vi "Subversion Get Status.vi"() -> (0 "error out":errorcluster, 1 "Working copy URL":string, 2 "Last \"Updated\" Date?":string, 3 "SVN Status":string)   [LabVIEW 2023]
uses:
  <vilib>/Utility/error.llb/Trim Whitespace One-Sided.vi
  <vilib>/regexp/Match Regular Expression.xnode
panel:
  out "Inhomogeneous revision?":bool
  out "Revision range if inhomogeneous":string
  out "Working copy uncommitted?":bool
  out "All Changed Files":string="0"
  out "Last Revision Different?":bool
  out "Last Revision":i32
  out "Revision":i32
  out "svn info":string
  out "Application Top-Level":path
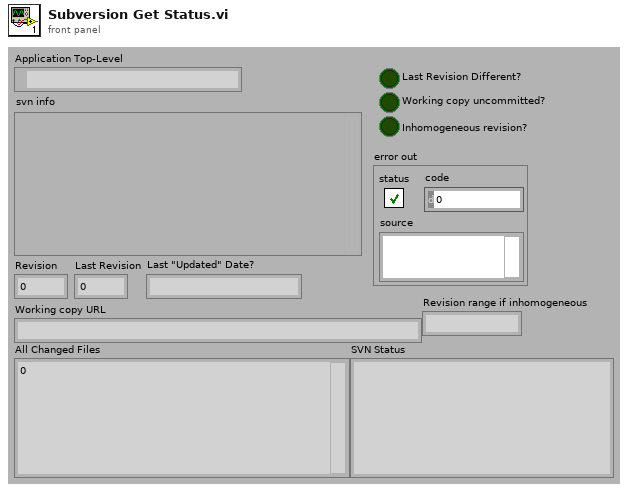
[diagram p1: front panel]
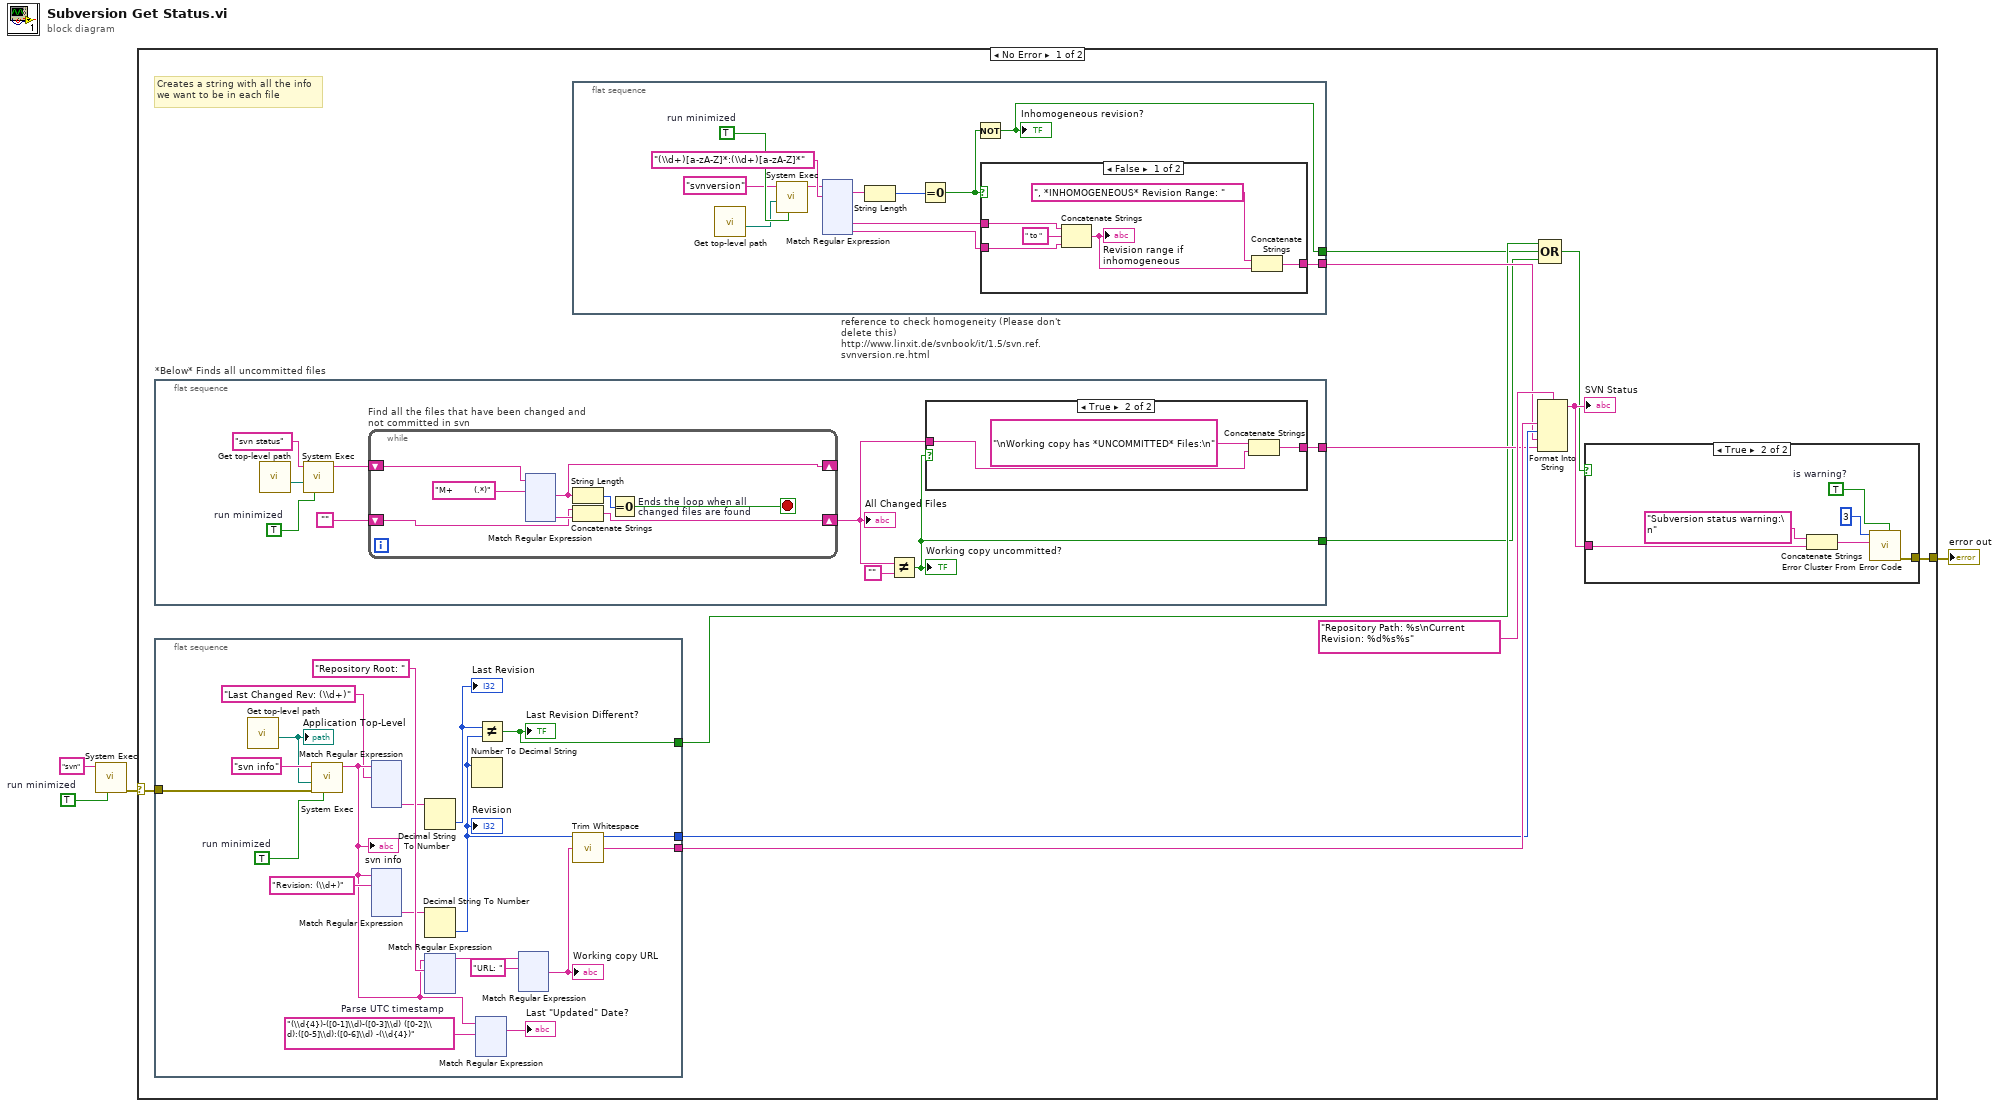
[diagram p0: block diagram]
diagram:
  w2 = TRUE  # run minimized
  n1 = call <vilib>:"System Exec.vi"("run minimized? (F)"=w2, "command line"="svn") -> ("error out"=w4:errorcluster)  [unwired: 4 in, 5 out]
  n2 = case shown="No Error" w4 {
    selector: w4 -> [w16 _]
    tunnel: [w5 _] -> w1
    frame No Error {
      # "Creates a string with all the info\nwe want to be in each file"
      n3 = flat-sequence "*Below* Finds all uncommitted files" {
        tunnel: [w770] -> w11
        tunnel: [w772] -> w8
        frame #0 {
          w776 = TRUE  # run minimized
          n4 = call "Get top-level path.vi"() -> ("Top-level LabVIEW path"=w774:path)  [unwired: 11 out]
          n5 = call <vilib>:"System Exec.vi"("run minimized? (F)"=w776, "working directory"=w774, "command line"="svn status" ("string")) -> ("standard output"=w775:string)  [unwired: 3 in, 5 out]
          n6 = while "Find all the files that have been changed and not committed in svn" {
            shift-right: [w784] -> w771
            shift-left: "" -> [w783]
            shift-right: [w781] -> _
            shift-left: w775 -> [w782]
            stop <- w785 stop-if-true
            n7 = xnode "Match Regular Expression"("input string"=w782, "regular expression"="M+       (.*)") -> ("after match"=w781:string, "submatch 1"=w786:string)  [unwired: 2 in, 6 out]
            n8 = String Length(string=w781) -> (length=w787:i32)
            n9 = Concatenate Strings(w783, w786) -> (w784:string)
            n10 = Equal To 0? "Ends the loop when all \nchanged files are found"(x=w787) -> (x = 0?=w785:bool)
          }
          "All Changed Files" <- w771
          n11 = Not Equal?(x=w771, y="") -> (x != y?=w772:bool)
          "Working copy uncommitted?" <- w772
          n12 = case shown="True" w772 {
            tunnel: [_ w778] -> w770
            tunnel: w771 -> [_ w779]
            frame False {
            }
            frame True {
              n13 = Concatenate Strings("\nWorking copy has *UNCOMMITTED* Files:\n" ("string"), w779) -> (w778:string)
            }
          }
        }
      }
      n14 = flat-sequence {
        tunnel: w16 -> [w28]
        tunnel: [w24] -> w14
        tunnel: [w27] -> w13
        tunnel: [w23] -> w10
        frame #0 {
          w34 = "(\\d{4})-([0-1]\\d)-([0-3]\\d) ([0-2]\\d):([0-5]\\d):([0-6]\\d) -(\\d{4})"  # Parse UTC timestamp
          w40 = TRUE  # run minimized
          n15 = call "Get top-level path.vi"() -> ("Top-level LabVIEW path"=w26:path)  [unwired: 11 out]
          "Application Top-Level" <- w26
          n16 = call <vilib>:"System Exec.vi"("run minimized? (F)"=w40, "error in (no error)"=w28, "working directory"=w26, "command line"="svn info" ("string")) -> ("standard output"=w32:string)  [unwired: 2 in, 5 out]
          "svn info" <- w32
          n17 = xnode "Match Regular Expression"("input string"=w32, "regular expression"="Last Changed Rev: (\\d+)") -> ("submatch 1"=w30:string)  [unwired: 2 in, 7 out]
          n18 = xnode "Match Regular Expression"("input string"=w32, "regular expression"="Revision: (\\d+)") -> ("submatch 1"=w35:string)  [unwired: 2 in, 7 out]
          n19 = Decimal String To Number(string=w30) -> (number=w29:i32)  [unwired: 3 out]
          "Last Revision" <- w29
          n20 = Decimal String To Number(string=w35) -> (number=w27:i32)  [unwired: 3 out]
          "Revision" <- w27
          n21 = xnode "Match Regular Expression"("input string"=w32, "regular expression"="Repository Root: ") -> ("before match"=w37:string)  [unwired: 2 in, 6 out]
          n22 = Number To Decimal String(number=w27) -> ()  [unwired: 2 out]
          n23 = xnode "Match Regular Expression"("input string"=w32, "regular expression"=w34) -> ("whole match"=→"Last \"Updated\" Date?":string)  [unwired: 2 in, 6 out]
          n24 = Not Equal?(x=w29, y=w27) -> (x != y?=w23:bool)
          "Last Revision Different?" <- w23
          n25 = xnode "Match Regular Expression"("input string"=w37, "regular expression"="URL: ") -> ("after match"=w25:string)  [unwired: 2 in, 6 out]
          "Working copy URL" <- w25
          n26 = call <vilib>:"Trim Whitespace.vi"("string"=w25) -> ("trimmed string"=w24:string)  [unwired: 1 in]
        }
      }
      n27 = flat-sequence "reference to check homogeneity (Please don't delete this)\nhttp://www.linxit.de/svnbook/it/1.5/svn.ref.svnversion.re.html" {
        tunnel: [w633] -> w12
        tunnel: [w631] -> w9
        frame #0 {
          w642 = TRUE  # run minimized
          n28 = call "Get top-level path.vi"() -> ("Top-level LabVIEW path"=w632:path)  [unwired: 11 out]
          n29 = call <vilib>:"System Exec.vi"("run minimized? (F)"=w642, "working directory"=w632, "command line"="svnversion" ("string")) -> ("standard output"=w634:string)  [unwired: 3 in, 5 out]
          n30 = xnode "Match Regular Expression"("input string"=w634, "regular expression"="(\\d+)[a-zA-Z]*:(\\d+)[a-zA-Z]*") -> ("whole match"=w638:string, "submatch 1"=w637:string, "submatch 2"=w636:string)  [unwired: 2 in, 6 out]
          n31 = String Length(string=w638) -> (length=w640:i32)
          n32 = Equal To 0?(x=w640) -> (x = 0?=w635:bool)
          n33 = Not(x=w635) -> (.not. x?=w631:bool)
          "Inhomogeneous revision?" <- w631
          n34 = case shown="False" w635 {
            tunnel: w637 -> [w648 _]
            tunnel: w636 -> [w647 _]
            tunnel: [w644 _] -> w633
            frame False {
              n35 = Concatenate Strings(w648, " to " ("string"), w647) -> (w645:string)
              "Revision range if inhomogeneous" <- w645
              n36 = Concatenate Strings(", *INHOMOGENEOUS* Revision Range: ", w645) -> (w644:string)
            }
            frame True {
            }
          }
        }
      }
      n37 = Format Into String(format string="Repository Path: %s\nCurrent Revision: %d%s%s", w14, w13, w12, w11) -> (resulting string=w7:string)  [unwired: 2 in, 1 out]
      "SVN Status" <- w7
      n38 = Compound Arithmetic op=OR(w10, w9, w8) -> (w6:bool)
      n39 = case shown="True" w6 {
        tunnel: w7 -> [_ w18]
        tunnel: [_ w17] -> w5
        frame False {
        }
        frame True {
          w22 = TRUE  # is warning?
          n40 = Concatenate Strings("Subversion status warning:\n" ("string"), w18) -> (w20:string)
          n41 = call <vilib>:"Error Cluster From Error Code.vi"("is warning? (False)"=w22, "error message (\"\")"=w20, "error code (0)"=3) -> ("error out"=w17:errorcluster)  [unwired: 2 in, 4 out]
        }
      }
    }
    frame Error {
    }
  }
  "error out" <- w1
